vi "WriteDictionary - private.vi"(8 "error in (no error)":errorcluster, 10 "Localization":T1, 11 "Dictionary Path":path) -> (0 "error out":errorcluster, 2 "JSON String":string, 3 "Dictionary Path Dup":path)   [LabVIEW 2017, in "JKI Simple Localization.lvlib"]
uses:
  API/JKI Simple Localization.lvlib
  Definitions/Dictionary--Cluster.ctl
  Definitions/Private/FontCluster.ctl
  Definitions/Private/Phrase Dictionary.ctl
  <vilib>/addons/_JKI.lib/Serialization/JSON/JKI JSON Serialization.lvlib
panel:
  # "{\n    \"Languages\":[\n        \"English\",\n        \"Dutch\",\n        \"Chinese\"\n    ],\n    \"Fonts\":[\n        {\n            \"Language\":\"English\",\n            \"Name\":\"Roboto Light\",\n            \"Color\":3947580\n        },\n        {\n            \"Language\":\"Dutch\",\n            \"Name\":\"Roboto Light\",\n            \"Color\":3947580\n        },\n        {\n            \"Language\":\"Chinese\",\n            \"Name\":\"SimSun\",\n            \"Color\":3947580\n        }\n    ],\n    \"Phrase Dictionary\":[\n        {\n            \"Key\":\"Language ListBox.Item0\",\n            \"Phrases\":[\n                \"English\",\n                \"Engels\",\n                \"英语\"\n            ]\n        },\n        {\n            \"Key\":\"Language ListBox.Item1\",\n            \"Phrases\":[\n                \"Dutch\",\n                \"Nederlands\",\n                \"荷兰人\"\n            ]\n        },\n        {\n            \"Key\":\"Language ListBox.Item2\",\n            \"Phrases\":[\n                \"Chinese\",\n                \"Chinese\",\n                \"中文\"\n            ]\n        },\n        {\n            \"Key\":\"Language ListBox\",\n            \"Phrases\":[\n                \"Language\",\n                \"Taal\",\n                \"语言\"\n            ]\n        },\n        {\n            \"Key\":\"Data.Display.xAxisLabel\",\n            \"Phrases\":[\n                \"Time (sec)\",\n                \"Tijd (sec)\",\n                \"时间（秒\"\n            ]\n        },\n        {\n            \"Key\":\"Data.Display.yAxisLabel\",\n            \"Phrases\":[\n                \"Voltage (V)\",\n                \"Voltage (V)\",\n                \"电压（V)\"\n            ]\n        },\n        {\n            \"Key\":\"Data.Display\",\n            \"Phrases\":[\n                \"Incoming Data\",\n                \"Inkomende Gegevens\",\n                \"传入数据\"\n            ]\n        },\n        {\n            \"Key\":\"Error.False\",\n            \"Phrases\":[\n                \"OFF\",\n                \"UIT\",\n                \"关闭\"\n            ]\n        },\n        {\n            \"Key\":\"Error.True\",\n            \"Phrases\":[\n                \"ON\",\n                \"AAN\",\n                \"上\"\n            ]\n        },\n        {\n            \"Key\":\"Error\",\n            \"Phrases\":[\n                \"Error\",\n                \"Fout\",\n                \"错误\"\n            ]\n        },\n        {\n            \"Key\":\"CustomControl.Increment.False\",\n            \"Phrases\":[\n                \"Okay\",\n                \"Oke\",\n                \"好的\"\n            ]\n        },\n        {\n            \"Key\":\"CustomControl.Increment.True\",\n            \"Phrases\":[\n                \"+1\",\n                \"+1\",\n                \"+1\"\n            ]\n        },\n        {\n            \"Key\":\"CustomControl.Increment\",\n            \"Phrases\":[\n                \"Increment\",\n                \"Nam Toe\",\n                \"增量\"\n            ]\n        },\n        {\n            \"Key\":\"Count\",\n            \"Phrases\":[\n                \"Count\",\n                \"Tel\",\n                \"伯爵\"\n            ]\n        },\n        {\n            \"Key\":\"Exit\",\n            \"Phrases\":[\n                \"Exit\",\n                \"Verlaten\",\n                \"出口\"\n            ]\n        },\n        {\n            \"Key\":\"Exit.BoolText\",\n            \"Phrases\":[\n                \"Exit\",\n                \"Verlaten\",\n                \"出口\"\n            ]\n        },\n        {\n            \"Key\":\"DialogText\",\n            \"Phrases\":[\n                \"This is an example of a localized string value.\",\n                \"Dit is een voorbeeld van een gelokaliseerde tekenreekswaarde\",\n                \"这是一个本地化字符串值的例子\"\n            ]\n        },\n        {\n            \"Key\":\"DialogConfirmation\",\n            \"Phrases\":[\n                \"Okay\",\n                \"Oke\",\n                \"好的\"\n            ]\n        },\n        {\n            \"Key\":\"Show Dialog\",\n            \"Phrases\":[\n                \"Show Localized Dialog\",\n                \"Toon gelokaliseerde dialoog\",\n                \"显示本地化对话\"\n            ]\n        },\n        {\n            \"Key\":\"Show Dialog.BoolText\",\n            \"Phrases\":[\n                \"Show\",\n                \"Toon\",\n                \"显示\"\n            ]\n        }\n    ]\n}"
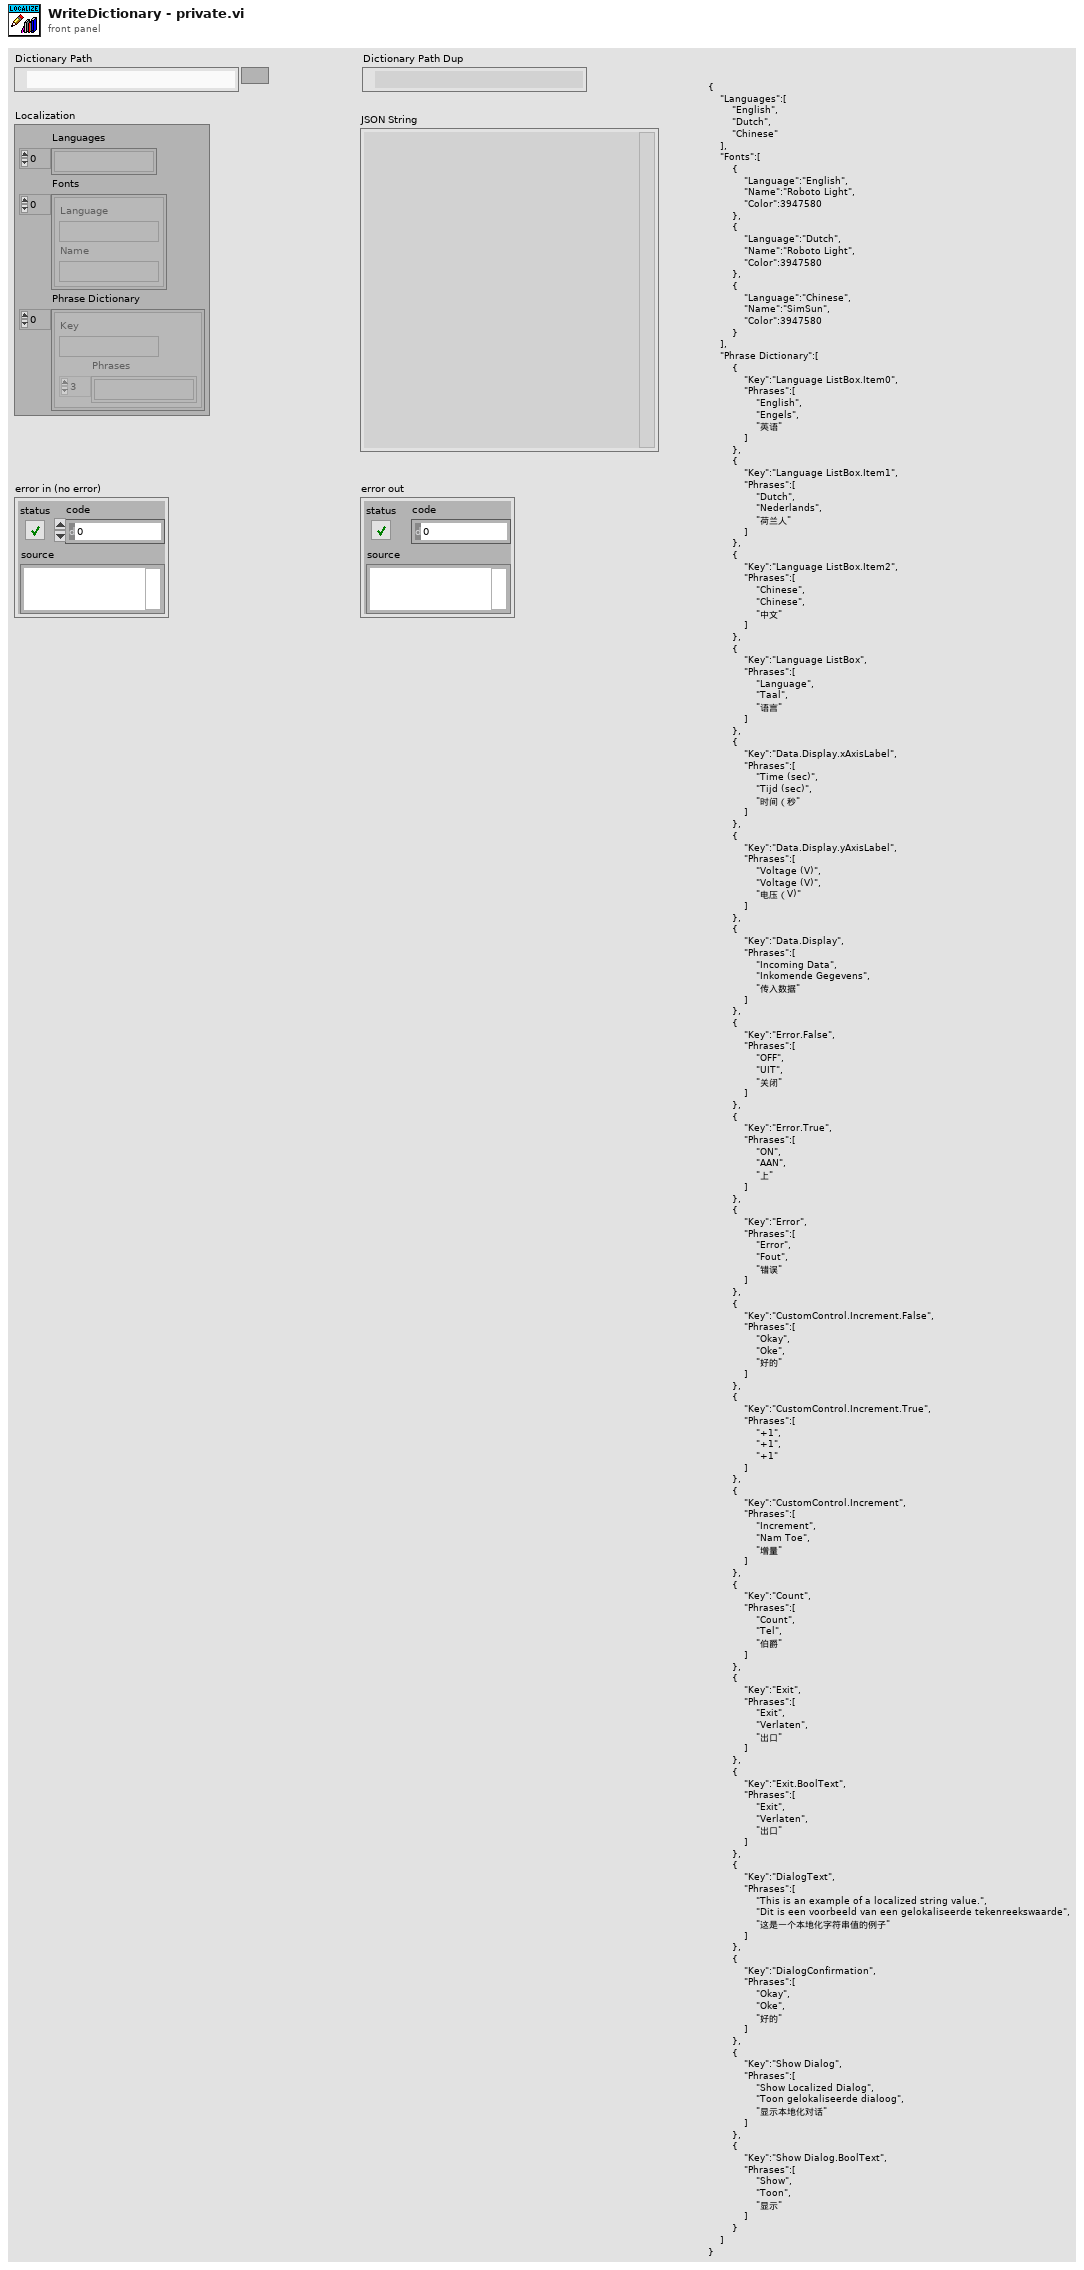
[diagram p1: front panel]
types:
  T1 = typedef "JKI Simple Localization.lvlib/Dictionary--Cluster.ctl" = cluster{"Languages":string[], "Fonts":T2[], "Phrase Dictionary":T3[]}
  T2 = typedef "JKI Simple Localization.lvlib/FontCluster.ctl" = cluster{"Language":string, "Name":string}
  T3 = typedef "JKI Simple Localization.lvlib/Phrase Dictionary.ctl" = cluster{"Key":string, "Phrases":string[]}
  T4 = enum16{"open", "replace", "create", "open or create", "replace or create", "replace or create with confirmation"}
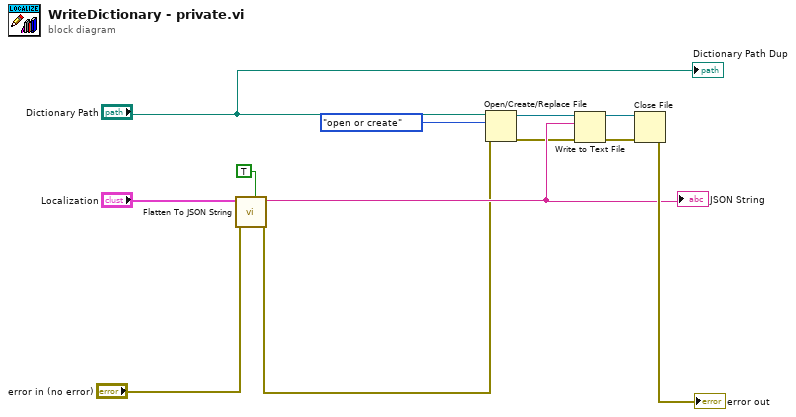
[diagram p0: block diagram]
diagram:
  n1 = call <vilib>:"Flatten To JSON String.vi"("Numeric Extensions (F)"=TRUE, "error in (no error)"="error in (no error)", "Variant"="Localization") -> ("error out"=w7:errorcluster, "JSON String"=w8:string)  [unwired: 7 in]
  "JSON String" <- w8
  n2 = Open/Create/Replace File(file path (use dialog)="Dictionary Path", error in=w7, operation (0:open)=T4."open or create") -> (refnum out=w2:refnum<file>, error out=w1:errorcluster)  [unwired: 3 in, 1 out]
  n3 = Write to Text File(file (use dialog)=w2, text=w8, error in=w1) -> (refnum out=w3:refnum<file>, error out=w4:errorcluster)  [unwired: 1 in, 1 out]
  n4 = Close File(refnum=w3, error in=w4) -> (error out=→"error out":errorcluster)  [unwired: 1 out]
  "Dictionary Path Dup" <- "Dictionary Path"
